vi "detector_get_data_dimensions.vi"(8 "error in (no error)":errorcluster, 11 "picoharp in":refnum<class "picoharp.lvclass">) -> (0 "error out":errorcluster, 1 "data_type":T1, 2 "dims":u32[](array[numeric]), 3 "picoharp out":refnum<class "picoharp.lvclass">)   [LabVIEW 2015, in "picoharp.lvclass"]
uses:
  picoharp.lvclass
  detector/data_types_tdef.ctl
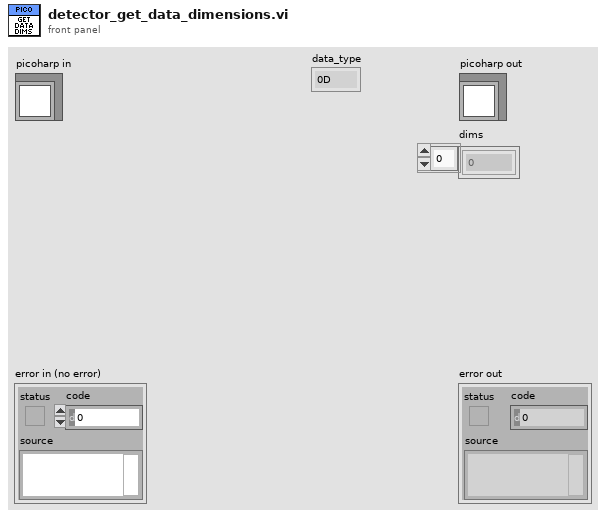
[diagram p1: front panel]
types:
  T1 = typedef "data_types_tdef.ctl" = enum16{"0D", "1D", "2D"}
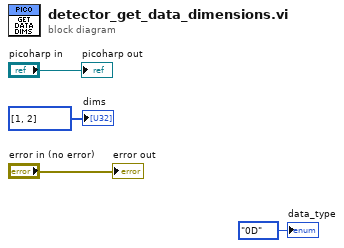
[diagram p0: block diagram]
diagram:
  "error out" <- "error in (no error)"
  "picoharp out" <- "picoharp in"
  "dims" <- u32[] [1, 2] ("dims")
  "data_type" <- data_types_tdef."0D" ("data_type")
